vi "testSelectState(s)Error_Error.vi"(8 "error in (no error)":errorcluster, 11 "testStateMachineUtilities in":refnum<class "testStateMachineUtilities.lvclass">) -> (0 "error out":errorcluster, 3 "testStateMachineUtilities out":refnum<class "testStateMachineUtilities.lvclass">)   [LabVIEW 2013, in "testStateMachineUtilities.lvclass"]
uses:
  testStateMachineUtilities.lvclass
  source/State Machine Support API/Select State(s)_err.vi
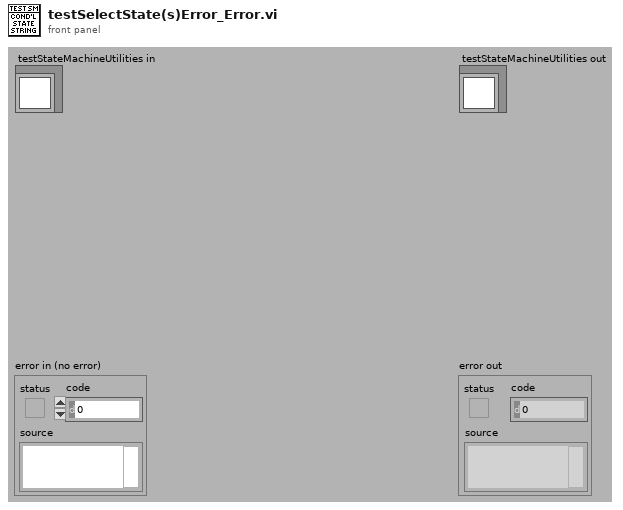
[diagram p1: front panel]
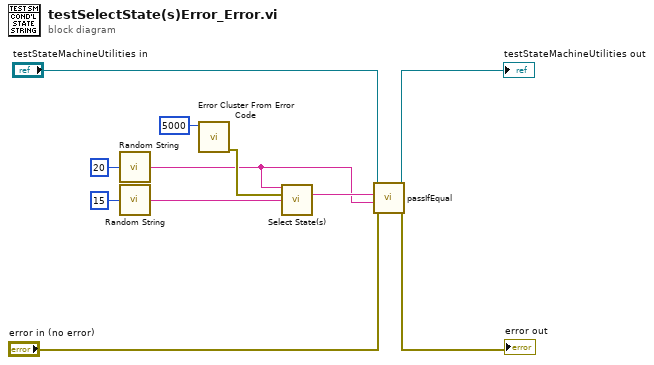
[diagram p0: block diagram]
diagram:
  n1 = call "Random String.vi"("Length"=20) -> ("ASCII"=w1:string)  [unwired: 4 in]
  n2 = call "Random String.vi"("Length"=15) -> ("ASCII"=w4:string)  [unwired: 4 in]
  n3 = call <vilib>:"Error Cluster From Error Code.vi"("error code (0)"=5000) -> ("error out"=w2:errorcluster)  [unwired: 8 in]
  n4 = call-poly "Select State(s).vi"("State(s) if True (\"\")"=w1, "Select"=w2, "State(s) if False (\"\")"=w4) -> ("States Out"=w5:string)  [unwired: 12 in]
  n5 = call-dynamic "passIfEqual.vi"("error in (no error)"="error in (no error)", "y"=w1, "x"=w5, "TestCase in"="testStateMachineUtilities in") -> ("error out"=→"error out":errorcluster, "TestCase out"=→"testStateMachineUtilities out":refnum<class "testStateMachineUtilities.lvclass">)  [unwired: 6 in]
